vi "Check for duplicates in 2D array column.vi"(6 "CSV file path":path, 8 "error in (no error)":errorcluster, 9 "Data Input source (2D array)":T1(ring), 10 "CSV field (0-N)":i32, 11 "Array":string[][](array[string])) -> (0 "error out":errorcluster, 1 "line count":i32, 2 "Duplicates Count":i32, 3 "Got duplicates?":bool, 4 "Sorted array":string[][](array[string]), 5 "CSV file array":string[][](array[string]), 7 "Duplicate data":string[](array[string]))   [LabVIEW 2013]
uses:
  <vilib>/Utility/file.llb/Read From Spreadsheet File (string).vi
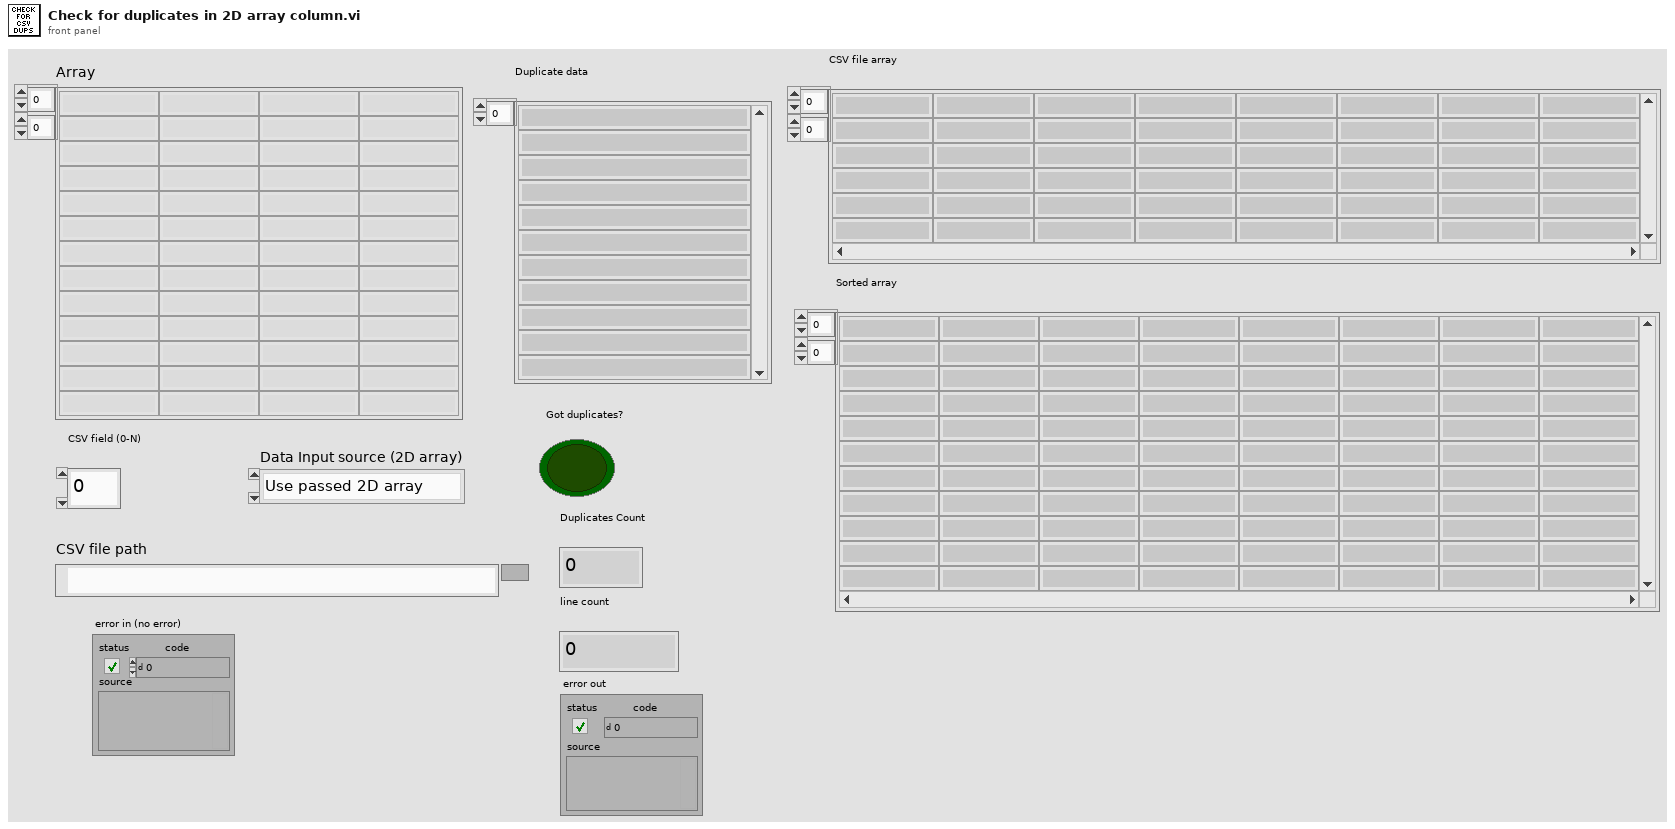
[diagram p1: front panel]
types:
  T1 = enum16{"Use passed 2D array", "Select CSV file", "Use passed file path"}
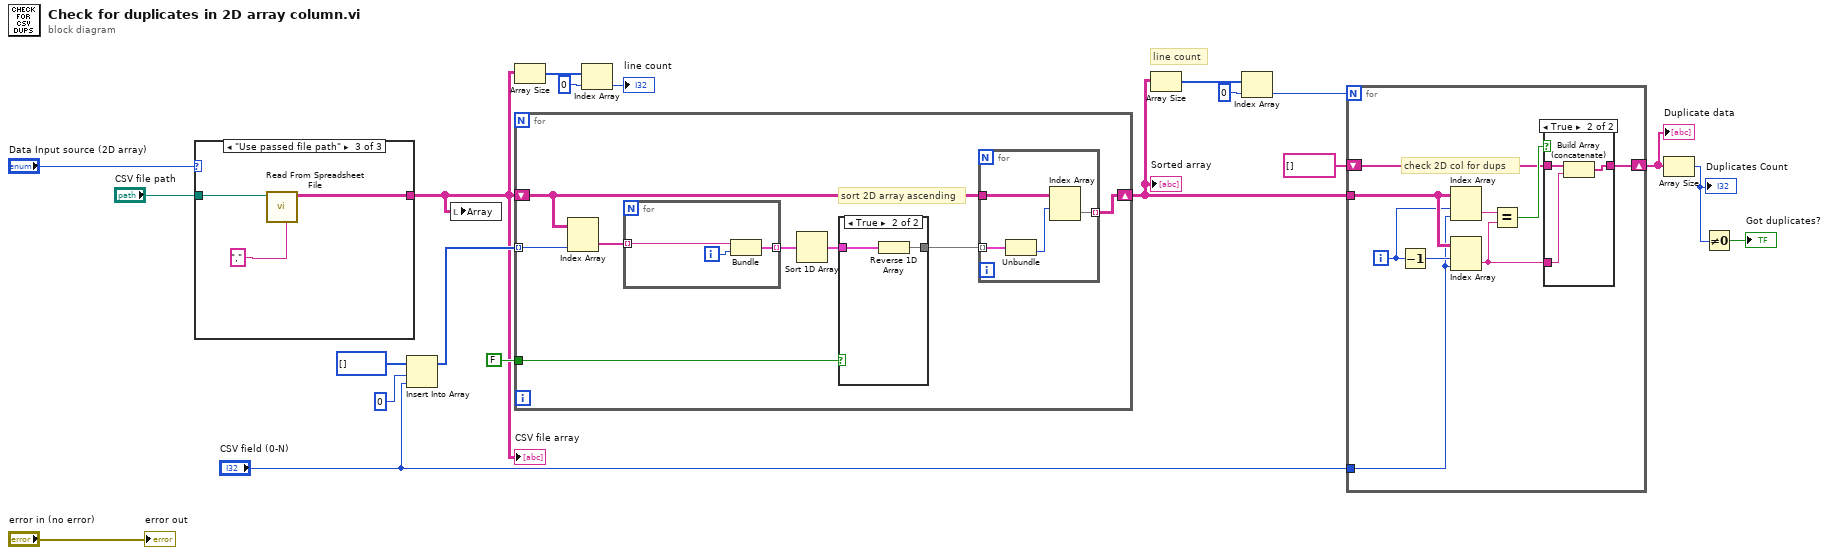
[diagram p0: block diagram]
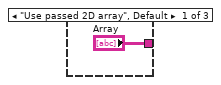
[diagram p3: hidden frame]
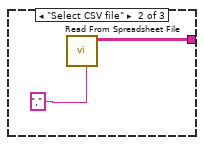
[diagram p4: hidden frame]
diagram:
  # "line count"
  n1 = case shown="\"Use passed file path\"" "Data Input source (2D array)" {
    tunnel: ["Array" w22 w24] -> w3
    tunnel: "CSV file path" -> [_ _ w25]
    frame "Use passed 2D array", Default {
    }
    frame "Select CSV file" {
      n2 = call-poly <vilib>:"Read From Spreadsheet File.vi"("delimiter (\\t)"="," ("delimiter (\\t)")) -> ("all rows"=w22:string[][])  [unwired: 6 in, 4 out]
    }
    frame "Use passed file path" {
      n3 = call-poly <vilib>:"Read From Spreadsheet File.vi"("delimiter (\\t)"="," ("delimiter (\\t)"), "file path (dialog if empty)"=w25) -> ("all rows"=w24:string[][])  [unwired: 5 in, 4 out]
    }
  }
  "CSV file array" <- w3
  n4 = Insert Into Array(array=i32[] [], index=0, new element="CSV field (0-N)") -> (w5:i32[])
  n5 = local write "Array"(w3) -> ()
  n6 = Array Size(array=w3) -> (size(s)=w20:i32[])
  n7 = for {
    shift-right: [w28] -> w2
    shift-left: w3 -> [w30]
    tunnel: w5 -> [w27] mode=indexing
    tunnel: FALSE ("Descending (F)") -> [w29]
    # "sort 2D array ascending"
    n8 = Index Array(array=w30, index (col)=w27) -> (element=w32:string[])  [unwired: 1 in]
    n9 = for {
      tunnel: w32 -> [w42] mode=indexing
      tunnel: [w44] -> w31 mode=indexing
      i -> [w43]
      n10 = Bundle("String"=w42, w43) -> (w44:cluster{"String":string, i32})  [unwired: 1 out]
    }
    n11 = Sort 1D Array(array=w31) -> (sorted array=w34:cluster{"String":string, i32}[])
    n12 = case shown="True" w29 {
      tunnel: [w35 w36] -> w33
      tunnel: w34 -> [w35 w37]
      frame False {
      }
      frame True {
        n13 = Reverse 1D Array(array=w37) -> (reversed array=w36:cluster{"String":string, i32}[])
      }
    }
    n14 = for {
      tunnel: w33 -> [w41] mode=indexing
      tunnel: w30 -> [w40]
      tunnel: [w38] -> w28 mode=indexing
      n15 = Unbundle(w41) -> (w39:i32)  [unwired: 1 out]
      n16 = Index Array(array=w40, index (row)=w39) -> (element=w38:string[])  [unwired: 1 in]
    }
  }
  "Sorted array" <- w2
  n17 = Index Array(array=w20, index=0) -> (element=→"line count":i32)
  n18 = Array Size(array=w2) -> (size(s)=w17:i32[])
  n19 = Index Array(array=w17, index=0) -> (element=w15:i32)
  n20 = for {
    N: w15 -> [_]
    tunnel: w2 -> [w53]
    tunnel: "CSV field (0-N)" -> [w50]
    shift-right: [w46] -> w13
    shift-left: string[] [] -> [w47]
    i -> [w52]
    # "check 2D col for dups"
    n21 = Decrement(x=w52) -> (x-1=w51:i32)
    n22 = Index Array(array=w53, index (row)=w52, index (col)=w50) -> (element=w49:string)
    n23 = Index Array(array=w53, index (row)=w51, index (col)=w50) -> (element=w45:string)
    n24 = Equal?(x=w49, y=w45) -> (x = y?=w48:bool)
    n25 = case shown="True" w48 {
      tunnel: w47 -> [w54 w57]
      tunnel: [w54 w55] -> w46
      tunnel: w45 -> [_ w56]
      frame False {
      }
      frame True {
        n26 = Build Array (concatenate)(w57, w56) -> (w55:string[])
      }
    }
  }
  "Duplicate data" <- w13
  n27 = Array Size(array=w13) -> (size(s)=w12:i32)
  "Duplicates Count" <- w12
  n28 = Not Equal To 0?(x=w12) -> (x != 0?=→"Got duplicates?":bool)
  "error out" <- "error in (no error)"
